vi "Cosmic Ray Processor.vi"(9 "Arbitrary Slope Shift":dbl=9001.0, 10 "Raw Data":i32[][](array[numeric]), 11 "Step Size":dbl=0.035) -> (2 "Processed Data":i32[][](array[numeric]), 3 "Cosmic Ray Location(s)":string)   [LabVIEW 2017]
doc: "Finds cosmic rays in raw data and replaces effected points with the average of its neighbors."
panel:
  out "Without":i32[](graph)
  out "Removed":dbl[](array[numeric])
  out "With 2":dbl[](array[numeric])
  out "With":i32[](graph)
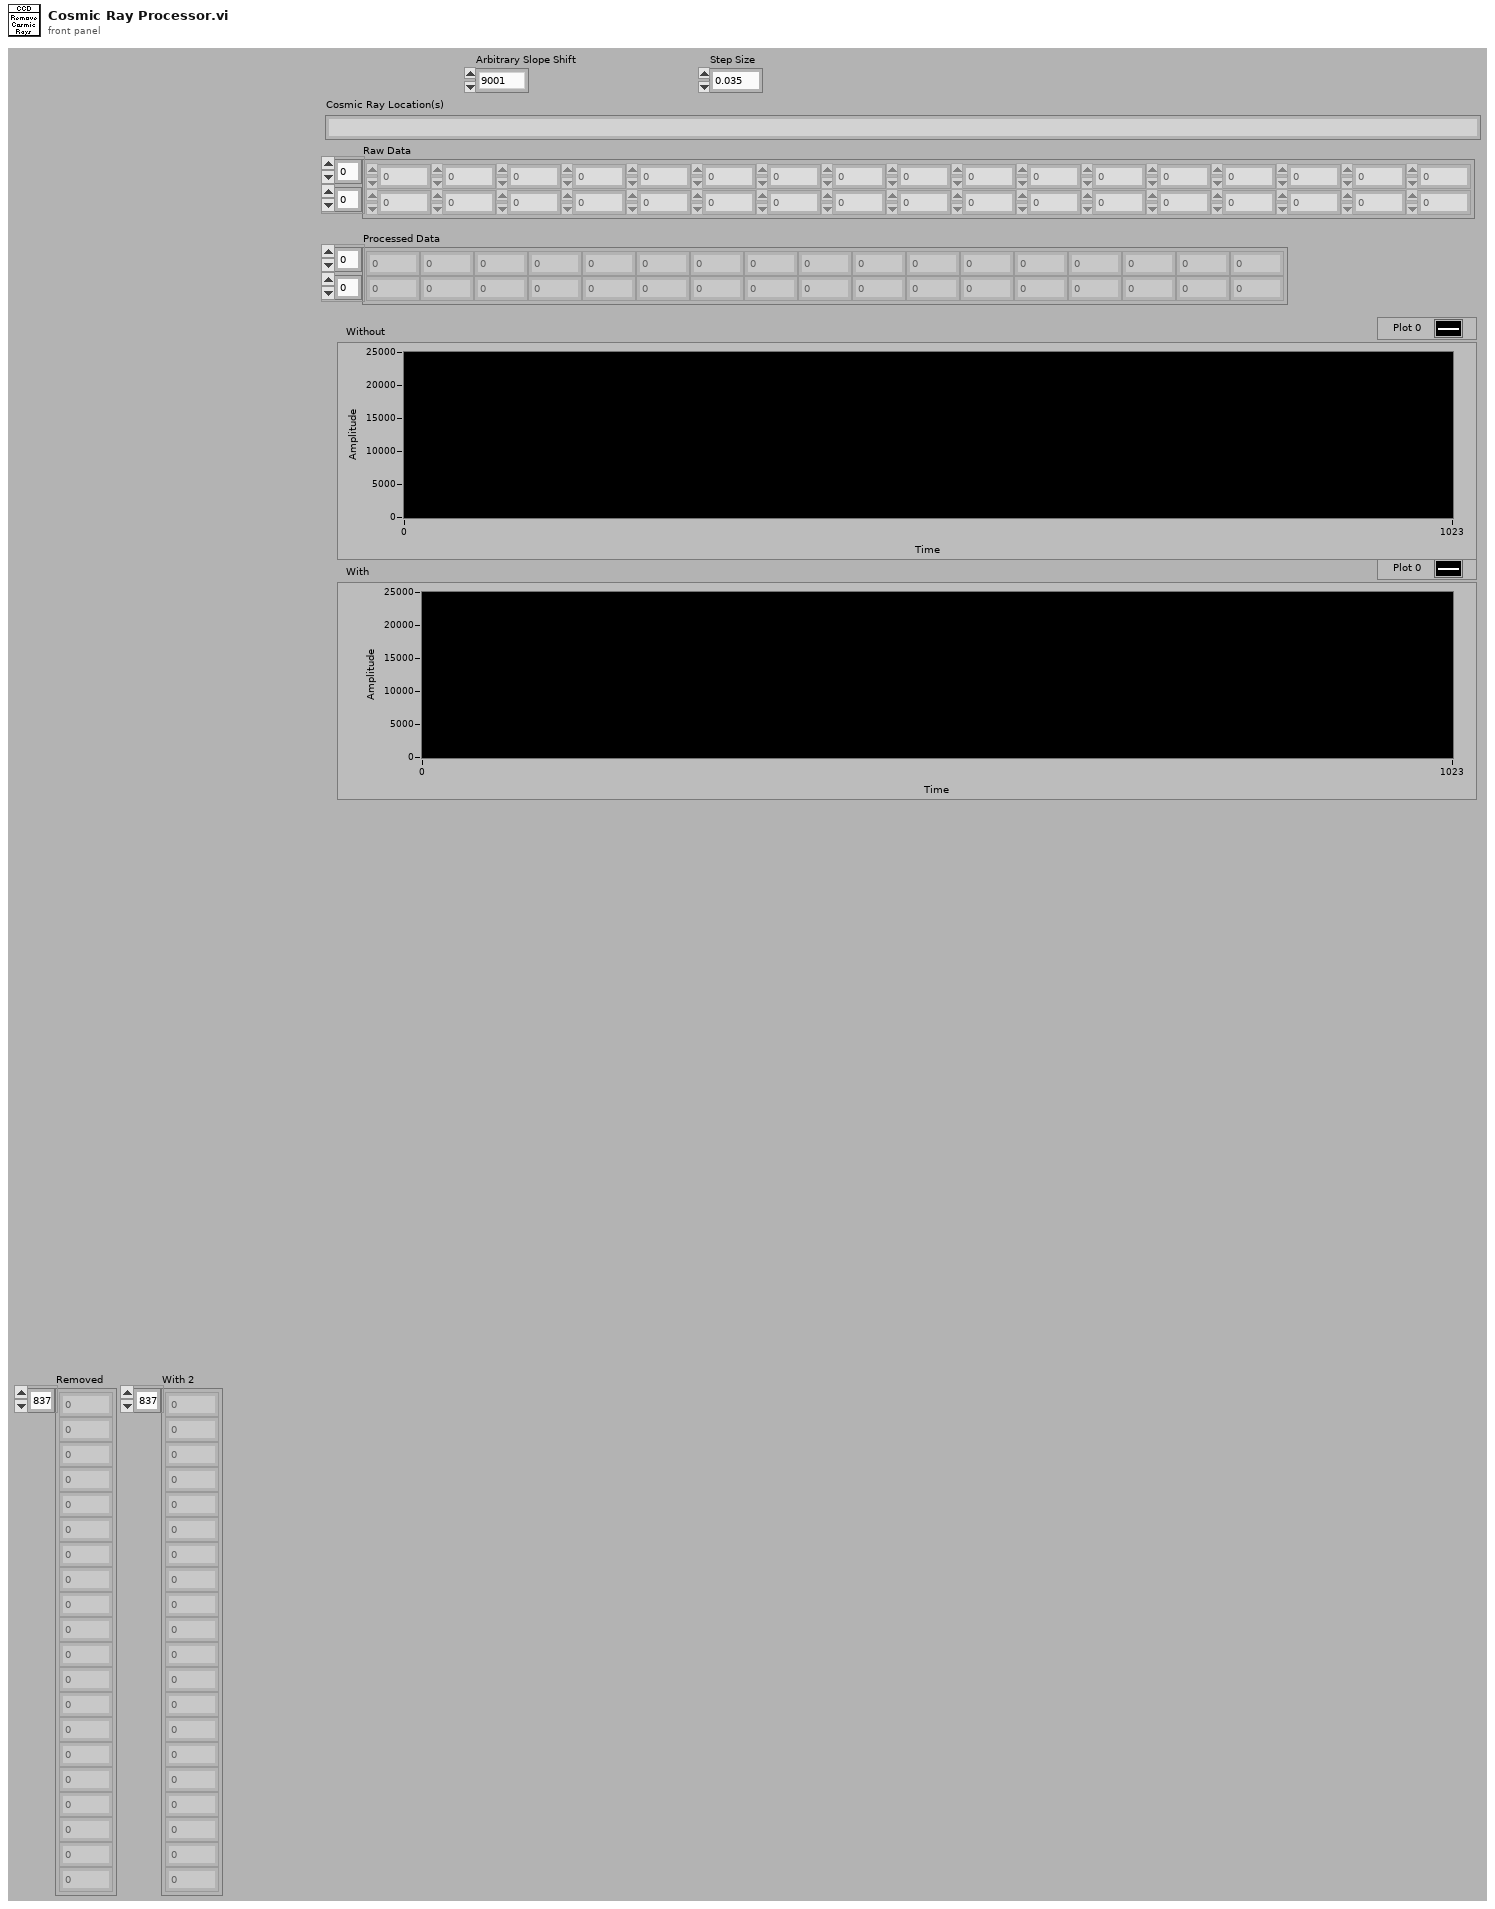
[diagram p1: front panel]
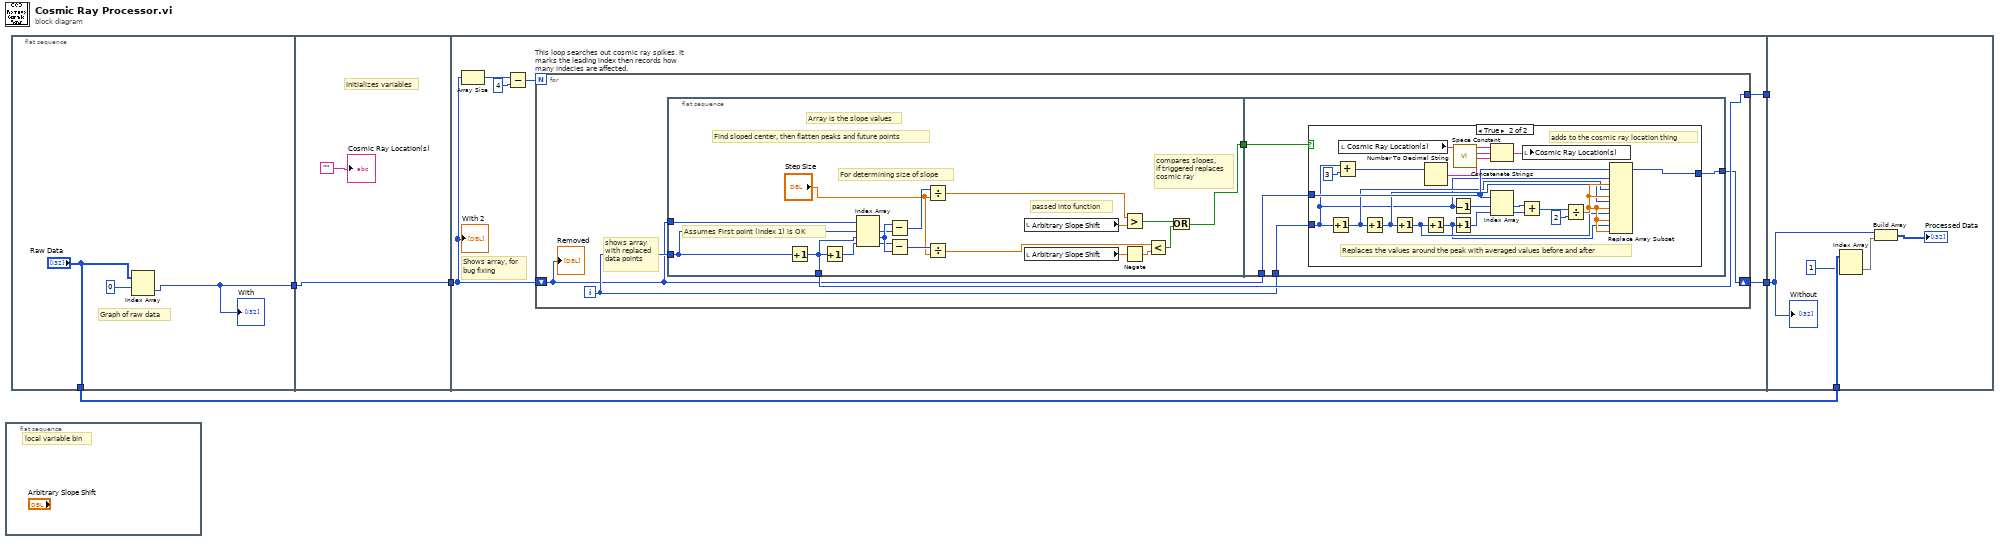
[diagram p0: block diagram]
diagram:
  n1 = flat-sequence {
    frame #0 {
      # "local variable bin"
    }
  }
  n2 = flat-sequence {
    tunnel: [w6] -> w5
    tunnel: ["Raw Data"] -> w1
    tunnel: [w9] -> w4
    tunnel: w5 -> [w9]
    tunnel: w4 -> [w12]
    tunnel: [w16] -> w3
    tunnel: [w11] -> w2
    tunnel: w3 -> [_]
    tunnel: w2 -> [w69]
    tunnel: w1 -> [w68]
    frame #0 {
      # "Graph of raw data"
      n3 = Index Array(array="Raw Data", index (row)=0) -> (element=w6:i32[])  [unwired: 1 in]
      "With" <- w6
    }
    frame #1 {
      # "Initializes variables"
      "Cosmic Ray Location(s)" <- ""
    }
    frame #2 {
      # "Shows array, for\nbug fixing"
      n4 = Array Size(array=w12) -> (size(s)=w15:i32)
      n5 = Subtract(x=w15, y=4) -> (x-y=w13:i32)
      n6 = for "This loop searches out cosmic ray spikes. It marks the leading index then records how many indecies are affected." {
        N: w13 -> [_]
        tunnel: [w21] -> w16
        shift-right: [w18] -> w11
        shift-left: w12 -> [w19]
        i -> [w20]
        # "shows array\nwith replaced\ndata points"
        n7 = flat-sequence {
          tunnel: [w29] -> w21
          tunnel: w20 -> [w31]
          tunnel: w19 -> [w32]
          tunnel: [w22] -> w17
          tunnel: w20 -> [w43]
          tunnel: w19 -> [w42]
          tunnel: [w41] -> w18
          tunnel: w17 -> [w40]
          frame #0 {
            # "compares slopes,\nif triggered replaces\ncosmic ray"
            # "passed into function"
            # "For determining size of slope"
            # "Array is the slope values"
            # "Find sloped center, then flatten peaks and future points"
            # "Assumes First point (index 1) is OK"
            n8 = Increment(x=w31) -> (x+1=w29:i32)
            n9 = Increment(x=w29) -> (x+1=w30:i32)
            n10 = Index Array(array=w32, index #1=w31, index #2=w29, index #3=w30) -> (element #1=w24:i32, element #2=w28:i32, element #3=w27:i32)
            n11 = Subtract(x=w28, y=w24) -> (x-y=w26:i32)
            n12 = Subtract(x=w27, y=w28) -> (x-y=w25:i32)
            n13 = Divide(x=w26, y="Step Size") -> (x/y=w34:dbl)
            n14 = Divide(x=w25, y="Step Size") -> (x/y=w33:dbl)
            n15 = local read "Arbitrary Slope Shift"() -> (w39:dbl)
            n16 = local read "Arbitrary Slope Shift"() -> (w38:dbl)
            n17 = Greater?(x=w34, y=w39) -> (0:w35:bool)
            n18 = Negate(x=w38) -> (-x=w37:dbl)
            n19 = Less?(x=w33, y=w37) -> (x < y?=w36:bool)
            n20 = Or(x=w35, y=w36) -> (x .or. y?=w22:bool)
          }
          frame #1 {
            n21 = case shown="True" w40 {
              tunnel: w43 -> [_ w46]
              tunnel: w42 -> [w44 w59]
              tunnel: [w44 w60] -> w41
              frame False {
              }
              frame True {
                # "Replaces the values around the peak with averaged values before and after"
                # "adds to the cosmic ray location thing"
                n22 = Increment(x=w46) -> (x+1=w52:i32)
                n23 = Add(x=w46, y=3) -> (x+y=w45:i32)
                n24 = local read "Cosmic Ray Location(s)"() -> (w64:string)
                n25 = Increment(x=w52) -> (x+1=w51:i32)
                n26 = Increment(x=w51) -> (x+1=w50:i32)
                n27 = Number To Decimal String(number=w45) -> (decimal integer string=w62:string)  [unwired: 1 in]
                n28 = Increment(x=w50) -> (x+1=w49:i32)
                n29 = Decrement(x=w46) -> (x-1=w56:i32)
                n30 = Increment(x=w49) -> (x+1=w48:i32)
                n31 = call <vilib>:"Space Constant.vi"() -> ("String"=w63:string)
                n32 = Concatenate Strings(w64, w63, w62) -> (w61:string)
                n33 = Index Array(array=w59, index #1=w56, index #2=w48) -> (element #1=w55:i32, element #2=w54:i32)
                n34 = Add(x=w55, y=w54) -> (x+y=w58:i32)
                n35 = local write "Cosmic Ray Location(s)"(w61) -> ()
                n36 = Divide(x=w58, y=2) -> (x/y=w53:dbl)
                n37 = Replace Array Subset(array=w59, new element #1=w53, index #1=w46, new element #2=w53, index #2=w52, new element #3=w53, index #3=w51, new element #4=w53, index #4=w50, new element #5=w53, index #5=w49) -> (w60:i32[])
              }
            }
          }
        }
        "Removed" <- w19
      }
      "With 2" <- w12
    }
    frame #3 {
      n38 = Index Array(array=w68, index (row)=1) -> (element=w66:i32[])  [unwired: 1 in]
      n39 = Build Array(w69, w66) -> (→"Processed Data":i32[][])
      "Without" <- w69
    }
  }
